vi "gloglo.vi"() -> ()   [LabVIEW 2020, in "UIA_UTsupport.lvlib" / "UIA_UTsupport.lvclass"]
uses:
  UIA_UTsupport.lvclass
panel:
  out "Latest DataString":string[](array[string])
  in  "AR Init counter":i32
  out "DIM SysLabels":string[](array[string])
  out "Latest Data":dbl[](array[numeric])
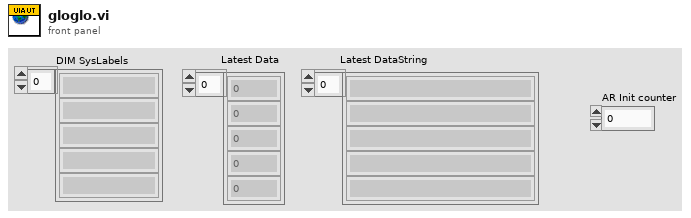
[diagram p1: front panel]
diagram:
